vi "Send Channel Settings.vi"(6 "Value to Send":T1, 8 "error in (no error)":errorcluster, 10 "Channel List":T2, 11 "3300 in":refnum<class "3300.lvclass">) -> (0 "error out":errorcluster, 3 "3300 out":refnum<class "3300.lvclass">)   [LabVIEW 2019]
uses:
  builds/Instruments/Electronic Load.lvlibp/Custom Controls/Channel Select.ctl
  builds/Instruments/Electronic Load.lvlibp/Parent/Custom Controls/Value to Send.ctl
  3300.lvclass
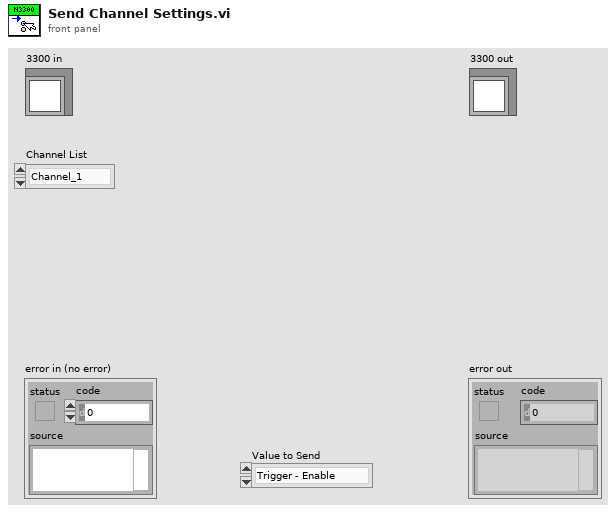
[diagram p1: front panel]
types:
  T1 = typedef "Electronic Load.lvlibp/Electronic Load.lvclass/Value to Send.ctl" = enum16{"Trigger - Enable", "Trigger - Sample Interval", "Trigger - Data Points", "Trigger - Current(Initial)", "Trigger - Transient Current", "Trigger - Pulse Width", "Trigger - Delay", "OCP - Enable", "OCP - Level", "OCP - Delay", "Function - Mode", "Function - Value", "Function - Enabled"}
  T2 = typedef "Electronic Load.lvlibp/Electronic Load.lvclass/Channel Select.ctl" = enum16{"Channel_1", "Channel_2", "Channel_3", "Channel_4", "Channel_5", "Channel_6"}
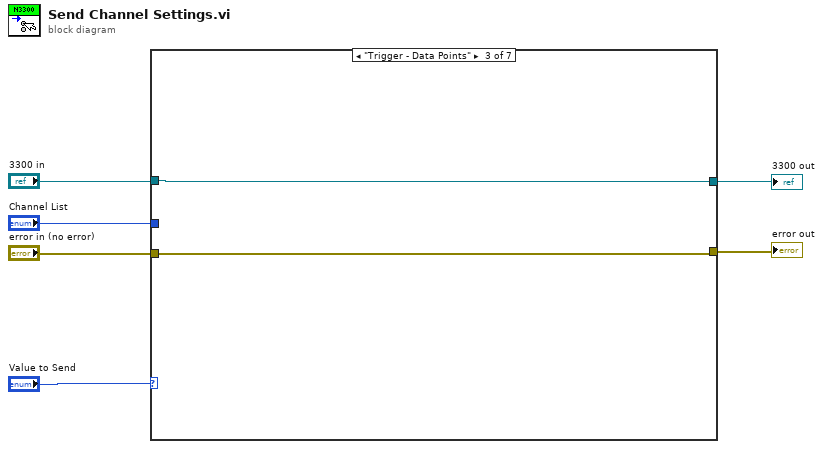
[diagram p0: block diagram]
diagram:
  n1 = case shown="\"Trigger - Data Points\"" "Value to Send" {
    tunnel: "3300 in" -> [w8 w10 w12 w14 w16 w18 w20]
    tunnel: [w8 w10 w12 w14 w16 w18 w20] -> w3
    tunnel: "error in (no error)" -> [w7 w9 w11 w13 w15 w17 w19]
    tunnel: [w7 w9 w11 w13 w15 w17 w19] -> w2
    tunnel: "Channel List" -> [_ _ _ _ _ _ _]
    frame "Trigger - Enable", Default {
    }
    frame "Trigger - Sample Interval" {
    }
    frame "Trigger - Data Points" {
    }
    frame "Trigger - Current(Initial)" {
    }
    frame "Trigger - Transient Current" {
    }
    frame "Trigger - Pulse Width" {
    }
    frame "Trigger - Delay" {
    }
  }
  "error out" <- w2
  "3300 out" <- w3
